vi "LoadRecordingscreen_171213.vi"(11 "Input":picture) -> (3 "Output":picture)   [LabVIEW 2016]
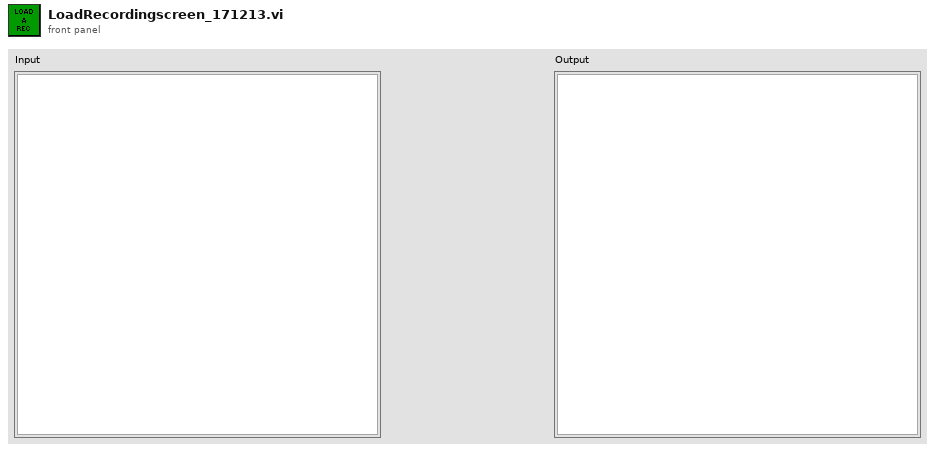
[diagram p1: front panel]
types:
  T1 = cluster{"Font Name:":string, "Size":i16, "Strikeout?":bool, "Italic?":bool, "Underline?":bool, "Outline?":bool, "Shadow?":bool, "Bold?":bool}
  T2 = enum16{"User-specified Font", "Application Font", "System Font", "Dialog Font"}
  T3 = enum16{"None", "Stacked", "Clockwise", "Counterclockwise"}
  T4 = cluster{"left":i16, "top":i16, "right":i16, "bottom":i16}
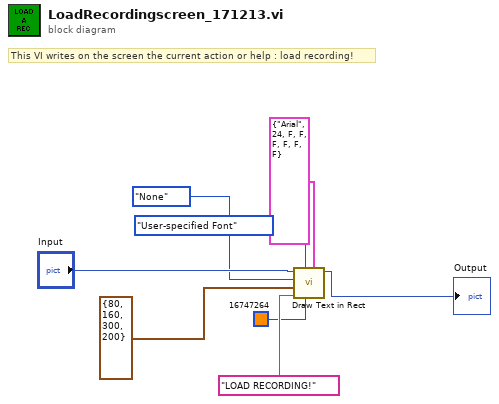
[diagram p0: block diagram]
diagram:
  # "This VI writes on the screen the current action or help : load recording!"
  n1 = call <vilib>:"Draw Text in Rect.vi"("[user-specified font]"=T1 {"Font Name:"="Arial", "Size"=24, "Strikeout?"=FALSE, "Italic?"=FALSE, "Underline?"=FALSE, "Outline?"=FALSE, "Shadow?"=FALSE, "Bold?"=FALSE}, "text color(black)"=u32 16747264, "desired font(Application)"=T2."User-specified Font", "text"="LOAD RECORDING!", "rect"=T4 {"left"=80, "top"=160, "right"=300, "bottom"=200}, "text orientation"=T3."None", "picture"="Input") -> ("new picture"=→"Output":picture)  [unwired: 4 in]
